vi "FPGA Download.vi"(8 "error in (no error)":errorcluster, 11 "FPGA Session In":refnum<class "FPGA Interface Base.lvclass">) -> (0 "error out":errorcluster, 3 "FPGA Session Out":refnum<class "FPGA Interface Base.lvclass">)   [LabVIEW 2010, in "FPGA Interface Base.lvclass"]
doc: "Re-downloads the FPGA bitstream to the target."
uses:
  <userlib>/_FPGA Interface Advanced Tools/FPGA Interface Base/FPGA Interface Base.lvclass
  <userlib>/_FPGA Interface Advanced Tools/FPGA Interface Base/Accessors/FPGA Read Session.vi
  <vilib>/Utility/error.llb/Error Cluster From Error Code.vi
  <userlib>/_FPGA Interface Advanced Tools/FPGA Interface Wrapper/FPGA Interface Wrapper.lvlib
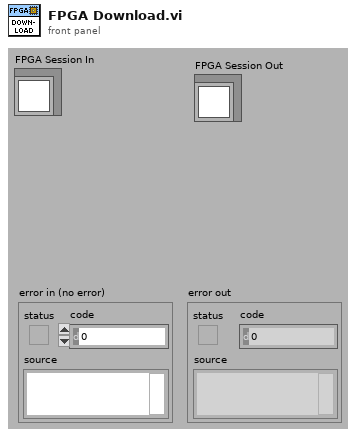
[diagram p1: front panel]
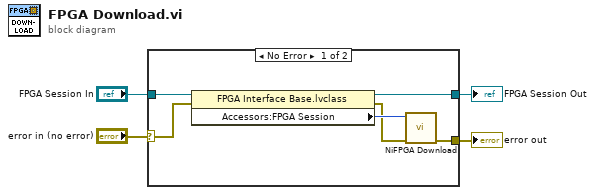
[diagram p0: block diagram]
diagram:
  n1 = case shown="No Error" "error in (no error)" {
    selector: "error in (no error)" -> [w9 w12]
    tunnel: [w5 w12] -> w1
    tunnel: [w6 w11] -> w3
    tunnel: "FPGA Session In" -> [w10 w11]
    frame No Error {
      n2 = property class="FPGA Interface Base.lvclass"(reference=w10, error in=w9) -> (reference out=w6:refnum<class "FPGA Interface Base.lvclass">, error out=w7:errorcluster, "Accessors:FPGA Session"=w8:u32)
      n3 = call <userlib>:"NiFPGA Download.vi"("error in (no error)"=w7, "Session"=w8) -> ("error out"=w5:errorcluster)  [unwired: 8 in, 1 out]
    }
    frame Error {
    }
  }
  "error out" <- w1
  "FPGA Session Out" <- w3
